vi "Auto indexing(for loop).vi"() -> ()   [LabVIEW 2018]
panel:
  out "Array 2":dbl[](array[numeric])
  out "Array":dbl[](array[numeric])
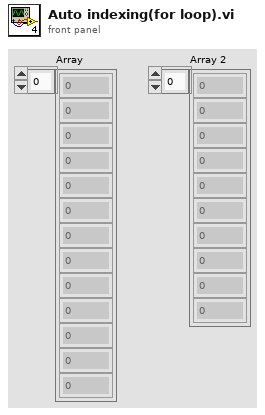
[diagram p1: front panel]
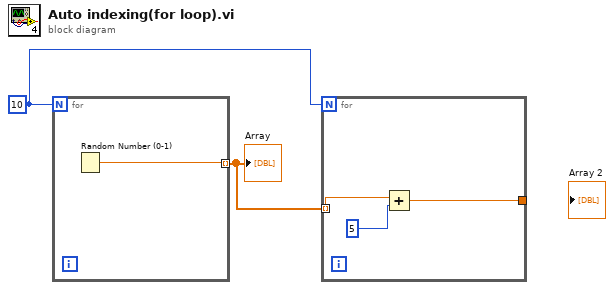
[diagram p0: block diagram]
diagram:
  w2 = 10
  n1 = for {
    N: w2 -> [_]
    tunnel: [w3] -> w1 mode=indexing
    n2 = Random Number (0-1)() -> (number: 0 to 1=w3:dbl)
  }
  "Array" <- w1
  n3 = for {
    N: w2 -> [_]
    tunnel: w1 -> [w6] mode=indexing
    tunnel: [w4] -> _
    n4 = Add(x=w6, y=5) -> (x+y=w4:dbl)
  }
